vi "DB Tools Get Types From DB.vi"(4 "error in (no error)":errorcluster, 6 "file?":bool, 7 "database":T1) -> (0 "error out":errorcluster, 3 "data types":string[](array[string]))   [LabVIEW 2017, in "NI_Database_API.lvlib"]
doc: "Returns the data types (array of strings) supported by the specified database or by the dbtypes.ini file."
uses:
  <vilib>/addons/database/NI_Database_API.lvlib
  <vilib>/addons/database/Auxilliary.llb/DB Tools Database.ctl
  <vilib>/addons/database/Auxilliary.llb/DB Tools SQL Server Types.ctl
  <vilib>/addons/database/Auxilliary.llb/DB Tools dBASE Types.ctl
  <vilib>/addons/database/Auxilliary.llb/DB Tools Jet Types.ctl
  <vilib>/addons/database/Auxilliary.llb/DB Tools Oracle Types.ctl
  <vilib>/addons/database/Auxilliary.llb/DB Tools MySQL Types.ctl
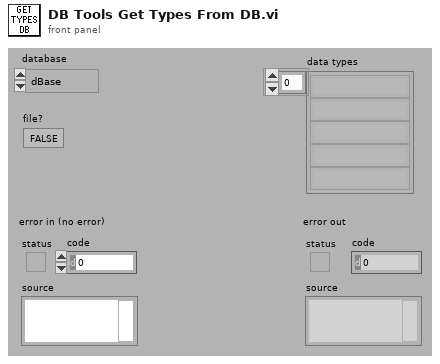
[diagram p1: front panel]
types:
  T1 = typedef "NI_Database_API.lvlib/DB Tools Database.ctl" = enum16{"dBase", "Jet", "SQL Server", "Oracle", "MySql"}
  T2 = typedef "NI_Database_API.lvlib/DB Tools SQL Server Types.ctl" = enum16{"varchar", "integer", "real", "float", "datetime", "image"}
  T3 = typedef "NI_Database_API.lvlib/DB Tools dBASE Types.ctl" = enum16{"varchar", "integer", "real", "float", "datetime", "oleobject"}
  T4 = typedef "NI_Database_API.lvlib/DB Tools Jet Types.ctl" = enum16{"varchar", "integer", "real", "float", "datetime", "oleobject"}
  T5 = typedef "NI_Database_API.lvlib/DB Tools Oracle Types.ctl" = enum16{"varchar", "integer", "real", "float", "date", "blob"}
  T6 = typedef "NI_Database_API.lvlib/DB Tools MySQL Types.ctl" = enum16{"varchar", "integer", "float", "double", "date", "blob"}
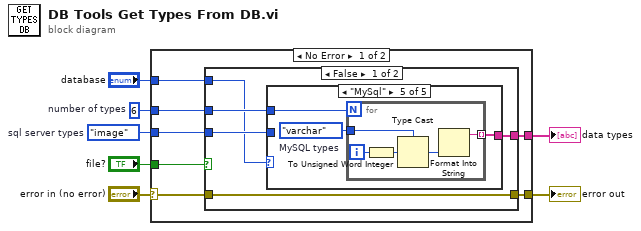
[diagram p0: block diagram]
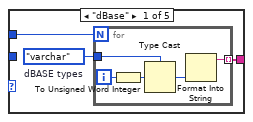
[diagram p2: hidden frame]
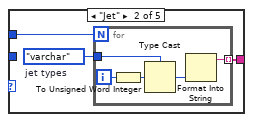
[diagram p3: hidden frame]
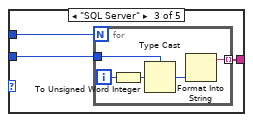
[diagram p4: hidden frame]
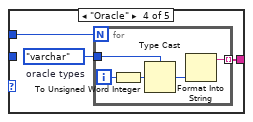
[diagram p5: hidden frame]
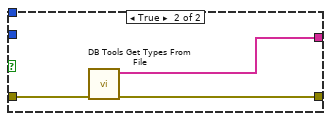
[diagram p6: hidden frame]
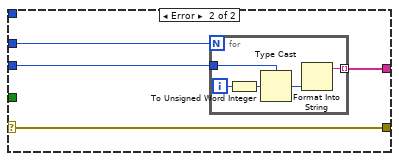
[diagram p7: hidden frame]
diagram:
  w4 = DB_Tools_SQL_Server_Types."image"  # sql server types
  w5 = 6  # number of types
  n1 = case shown="No Error" "error in (no error)" {
    selector: "error in (no error)" -> [w13 w66]
    tunnel: [w14 w66] -> w7
    tunnel: w5 -> [w12 w65]
    tunnel: w4 -> [w11 w64]
    tunnel: [w10 w63] -> w3
    tunnel: "database" -> [w9 _]
    tunnel: "file?" -> [w8 _]
    frame No Error {
      n2 = case shown="False" w8 {
        tunnel: w13 -> [w19 w62]
        tunnel: [w19 w61] -> w14
        tunnel: w12 -> [w18 _]
        tunnel: w11 -> [w16 _]
        tunnel: [w17 w60] -> w10
        tunnel: w9 -> [w15 _]
        frame False {
          n3 = case shown="\"MySql\"" w15 {
            tunnel: w18 -> [w22 w30 w38 w46 w53]
            tunnel: [w21 w29 w37 w45 w54] -> w17
            tunnel: w16 -> [_ _ w36 _ _]
            frame "dBase" {
              w20 = DB_Tools_dBASE_Types."varchar"  # dBASE types
              n4 = for {
                N: w22 -> [_]
                tunnel: [w24] -> w21 mode=indexing
                tunnel: w20 -> [w23]
                i -> [w27]
                n5 = To Unsigned Word Integer(number=w27) -> (unsigned 16bit integer=w26:u16)
                n6 = Type Cast(type=w23, x=w26) -> (*(type *) &x=w25:T3)
                n7 = Format Into String(w25) -> (resulting string=w24:string)  [unwired: 3 in, 1 out]
              }
            }
            frame "Jet" {
              w28 = DB_Tools_Jet_Types."varchar"  # jet types
              n8 = for {
                N: w30 -> [_]
                tunnel: [w32] -> w29 mode=indexing
                tunnel: w28 -> [w31]
                i -> [w35]
                n9 = To Unsigned Word Integer(number=w35) -> (unsigned 16bit integer=w34:u16)
                n10 = Type Cast(type=w31, x=w34) -> (*(type *) &x=w33:T4)
                n11 = Format Into String(w33) -> (resulting string=w32:string)  [unwired: 3 in, 1 out]
              }
            }
            frame "SQL Server" {
              n12 = for {
                N: w38 -> [_]
                tunnel: [w40] -> w37 mode=indexing
                tunnel: w36 -> [w39]
                i -> [w43]
                n13 = To Unsigned Word Integer(number=w43) -> (unsigned 16bit integer=w42:u16)
                n14 = Type Cast(type=w39, x=w42) -> (*(type *) &x=w41:T2)
                n15 = Format Into String(w41) -> (resulting string=w40:string)  [unwired: 3 in, 1 out]
              }
            }
            frame "Oracle" {
              w44 = DB_Tools_Oracle_Types."varchar"  # oracle types
              n16 = for {
                N: w46 -> [_]
                tunnel: [w48] -> w45 mode=indexing
                tunnel: w44 -> [w47]
                i -> [w51]
                n17 = To Unsigned Word Integer(number=w51) -> (unsigned 16bit integer=w50:u16)
                n18 = Type Cast(type=w47, x=w50) -> (*(type *) &x=w49:T5)
                n19 = Format Into String(w49) -> (resulting string=w48:string)  [unwired: 3 in, 1 out]
              }
            }
            frame "MySql" {
              w52 = DB_Tools_MySQL_Types."varchar"  # MySQL types
              n20 = for {
                N: w53 -> [_]
                tunnel: [w56] -> w54 mode=indexing
                tunnel: w52 -> [w55]
                i -> [w59]
                n21 = To Unsigned Word Integer(number=w59) -> (unsigned 16bit integer=w58:u16)
                n22 = Type Cast(type=w55, x=w58) -> (*(type *) &x=w57:T6)
                n23 = Format Into String(w57) -> (resulting string=w56:string)  [unwired: 3 in, 1 out]
              }
            }
          }
        }
        frame True {
          n24 = call <vilib>:"DB Tools Get Types From File.vi"("error in (no error)"=w62) -> ("error out"=w61:errorcluster, "data types"=w60:string[])  [unwired: 5 in]
        }
      }
    }
    frame Error {
      n25 = for {
        N: w65 -> [_]
        tunnel: [w68] -> w63 mode=indexing
        tunnel: w64 -> [w67]
        i -> [w71]
        n26 = To Unsigned Word Integer(number=w71) -> (unsigned 16bit integer=w70:u16)
        n27 = Type Cast(type=w67, x=w70) -> (*(type *) &x=w69:T2)
        n28 = Format Into String(w69) -> (resulting string=w68:string)  [unwired: 3 in, 1 out]
      }
    }
  }
  "error out" <- w7
  "data types" <- w3
